vi "Setup UI.vi"(8 "error in (no error)":errorcluster, 10 "Set UI to input? (F)":bool, 11 "Wavelength iHR320 in":refnum<class "Wavelength ActiveX.lvclass">) -> (0 "error out":errorcluster, 3 "Wavelength iHR320 out":refnum<class "Wavelength ActiveX.lvclass">)   [LabVIEW 2023, in "Wavelength ActiveX.lvclass"]
doc: "Scanner::Setup is a constructor that has no parameters and faces the user. The Factory calls this VI to let the user configure this Scanner. It is dynamically dispatched in order to let the user choose the type as well as the options of the scanner."
uses:
  Wavelength ActiveX.lvclass
  Wavelength ActiveX.lvclass/Wavelength ActiveX.ctl
panel:
  in  "Select Filter":i32(ring)=1 items=["Filter 1"=1, "Empty"=2, "Empty"=3, "Empty"=4, "Filter 2"=5, "Filter 3"=6]
  out "Current Filter":i32(ring)=1 items=["Filter 1"=1, "Empty"=2, "Empty"=3, "Empty"=4, "Filter 2"=5, "Filter 3"=6]
  out "Current Position":dbl[unit]
  in  "GoTo First Step":bool
  out "Current Grating":dbl
  out "Step Size":dbl[unit]
  in  "Exit Slit":dbl[unit]=0.001
  in  "Entrance Slit":dbl[unit]=0.001
  in  "Override":bool
  in  "Select Grating":u16(ring)=2 items=["1200"=1, "600"=2]
  in  "Front Exit":dbl[unit]
  in  "Front Entrance":dbl[unit]
  # "iHR 320 Wavelength"
  # "lines/mm"
  # "lines/mm"
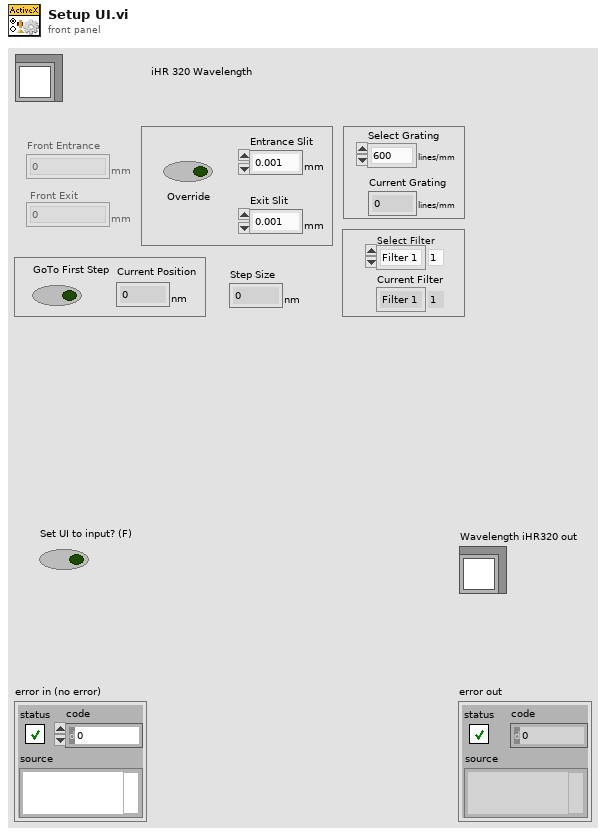
[diagram p1: front panel]
types:
  T1 = typedef "Scanner.lvclass/Range.ctl" = cluster{"xi":dbl, "xf":dbl, "dx":dbl, "Return to...?":bool, "Return to":dbl}
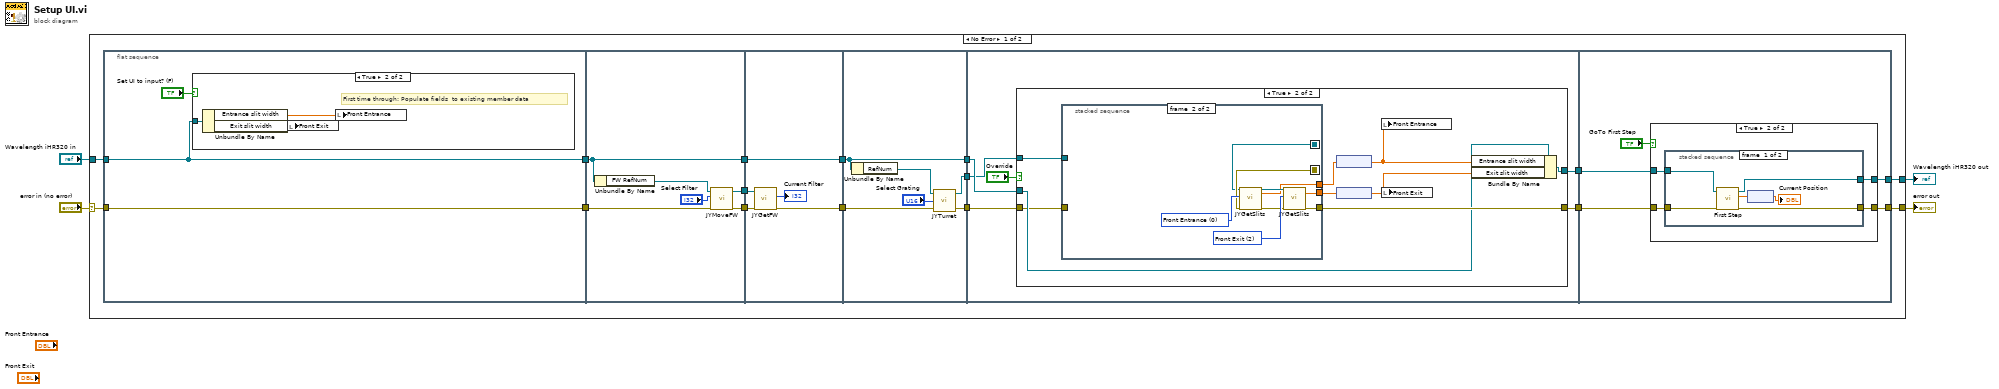
[diagram p0: block diagram]
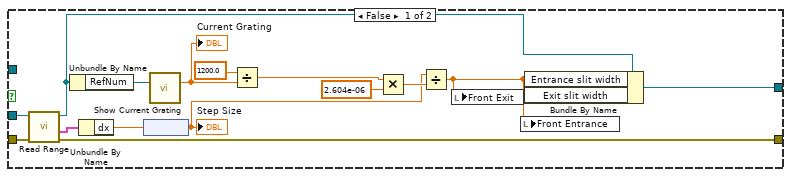
[diagram p3: hidden frame]
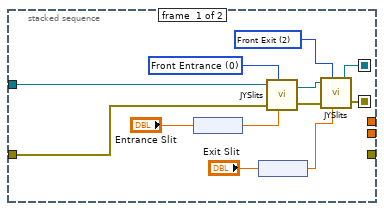
[diagram p4: hidden frame]
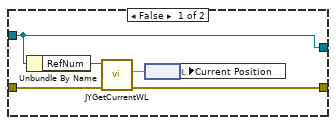
[diagram p5: hidden frame]
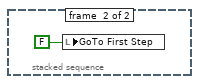
[diagram p6: hidden frame]
diagram:
  n1 = case shown="No Error" "error in (no error)" {
    selector: "error in (no error)" -> [w19 w118]
    tunnel: [w17 w118] -> w3
    tunnel: "Wavelength iHR320 in" -> [w20 w117]
    tunnel: [w18 w117] -> w1
    frame No Error {
      n2 = flat-sequence {
        tunnel: w20 -> [w21]
        tunnel: [w21] -> w12
        tunnel: [w22] -> w11
        tunnel: w19 -> [w22]
        tunnel: w12 -> [w29]
        tunnel: [w29] -> w10
        tunnel: w11 -> [w31]
        tunnel: [w30] -> w8
        tunnel: [w27] -> w6
        tunnel: w10 -> [w37]
        tunnel: [w37] -> w9
        tunnel: w8 -> [w35]
        tunnel: [w34] -> w7
        tunnel: w6 -> [w33]
        tunnel: w9 -> [w40]
        tunnel: w7 -> [w41]
        tunnel: [w40] -> w14
        tunnel: [w39] -> w13
        tunnel: [w38] -> w5
        tunnel: [w47] -> w16
        tunnel: [w48] -> w15
        tunnel: w14 -> [w46]
        tunnel: w13 -> [w45]
        tunnel: w5 -> [w44]
        tunnel: [w97] -> w17
        tunnel: [w96] -> w18
        tunnel: w16 -> [w99]
        tunnel: w15 -> [w98]
        frame #0 {
          n3 = case shown="True" "Set UI to input? (F)" {
            tunnel: w21 -> [_ w24]
            frame False {
              # "Subsequent times through: Populate member data  according to existing fields"
            }
            frame True {
              # "First time through: Populate fields  to existing member data"
              n4 = Unbundle By Name(w24) -> ("Entrance slit width"=w26:dbl[unit], "Exit slit width"=w25:dbl[unit])
              n5 = local write "Front Exit"(w25) -> ()
              n6 = local write "Front Entrance"(w26) -> ()
            }
          }
        }
        frame #1 {
          n7 = Unbundle By Name(w29) -> ("FW RefNum"=w28:refnum<k7>)
          n8 = call "JYMoveFW.vi"("error in (no error)"=w31, "Filter Index"="Select Filter", "FW RefNum In"=w28) -> ("error out"=w30:errorcluster, "FW RefNum Out"=w27:refnum<k7>)  [unwired: 7 in]
        }
        frame #2 {
          n9 = call "JYGetFW.vi"("error in (no error)"=w35, "FW RefNum In"=w33) -> ("error out"=w34:errorcluster, "Filter Index"=→"Current Filter":i32)  [unwired: 7 in, 1 out]
        }
        frame #3 {
          n10 = Unbundle By Name(w40) -> ("RefNum"=w42:refnum<k7>)
          n11 = call "JYTurret.vi"("error in (no error)"=w41, "Grating Index"="Select Grating", "JYMONOLib.IJYMonoReqd In"=w42) -> ("error out"=w39:errorcluster, "JYMONOLib.IJYMonoReqd Out"=w38:refnum<k7>)  [unwired: 1 out]
        }
        frame #4 {
          n12 = case shown="True" "Override" {
            tunnel: [w54 w73] -> w48
            tunnel: [w53 w72] -> w47
            tunnel: w46 -> [w51 w67]
            tunnel: w45 -> [w50 w66]
            tunnel: w44 -> [_ w65]
            frame False {
              n13 = call-dynamic "Read Range.vi"("error in (no error)"=w50, "Scanner.lvclass in"=w51) -> ("error out"=w54:errorcluster, "Range"=w52:T1, "Scanner.lvclass out"=w62:refnum<class "Wavelength ActiveX.lvclass">)  [unwired: 4 in, 3 out]
              n14 = Unbundle By Name(w62) -> ("RefNum"=w63:refnum<k7>)
              n15 = Unbundle By Name(w52) -> ("dx"=w64:dbl)
              n16 = node(w64) -> (w56:dbl[unit])
              "Step Size" <- w56
              n17 = call "Show Current Grating.vi"("JYMONOLib.IJYMonoReqd  in"=w63) -> ("Current Grating"=w60:dbl)  [unwired: 6 in, 8 out]
              "Current Grating" <- w60
              n18 = Divide(x=1200.0, y=w60) -> (x/y=w59:dbl)
              n19 = Multiply(x=w59, y=2.604e-06) -> (x*y=w57:dbl)
              n20 = Divide(x=w56, y=w57) -> (x/y=w55:dbl[unit])
              n21 = local write "Front Exit"(w55) -> ()
              n22 = local write "Front Entrance"(w55) -> ()
              n23 = Bundle By Name(cluster=w62, "Entrance slit width"=w55, "Exit slit width"=w55) -> (w53:refnum<class "Wavelength ActiveX.lvclass">)
            }
            frame True {
              n24 = stacked-sequence {
                seq-local: [w77 _] -> [_ w91]
                seq-local: [w74 _] -> [_ w86]
                tunnel: [_ w89] -> w73
                tunnel: [_ w88] -> w71
                tunnel: [_ w87] -> w70
                tunnel: w66 -> [w76 _]
                tunnel: w65 -> [w75 _]
                frame #0 {
                  w83 = u16 2 items=["Front Entrance", "Side Entrance", "Front Exit", "Side Exit", "First Intermediate", "Second Intermediate"] ("Slit")
                  w84 = u16 0 items=["Front Entrance", "Side Entrance", "Front Exit", "Side Exit", "First Intermediate", "Second Intermediate"] ("Slit")
                  n25 = node("Entrance Slit") -> (w85:dbl)
                  n26 = node("Exit Slit") -> (w82:dbl)
                  n27 = call "JYSlits.vi"("JYMONOLib.IJYMonoReqd In"=w75, "Slit"=w84, "error in (no error)"=w76, "Slit Width"=w85) -> ("JYMONOLib.IJYMonoReqd Out"=w81:refnum<k7>, "error out"=w80:errorcluster)  [unwired: 1 in]
                  n28 = call "JYSlits.vi"("JYMONOLib.IJYMonoReqd In"=w81, "Slit"=w83, "error in (no error)"=w80, "Slit Width"=w82) -> ("JYMONOLib.IJYMonoReqd Out"=w74:refnum<k7>, "error out"=w77:errorcluster)  [unwired: 1 in]
                }
                frame #1 {
                  w92 = u16 2 items=["Front Entrance", "Side Entrance", "Front Exit", "Side Exit", "First Intermediate", "Second Intermediate"] ("Slit")
                  w93 = u16 0 items=["Front Entrance", "Side Entrance", "Front Exit", "Side Exit", "First Intermediate", "Second Intermediate"] ("Slit")
                  n29 = call "JYGetSlits.vi"("MonoRefNum IN"=w86, "Slit"=w93, "error in (no error)"=w91) -> ("MonoRefNum Out"=w94:refnum<k7>, "Slit Width"=w88:dbl, "error out"=w90:errorcluster)  [unwired: 13 in, 1 out]
                  n30 = call "JYGetSlits.vi"("MonoRefNum IN"=w94, "Slit"=w92, "error in (no error)"=w90) -> ("Slit Width"=w87:dbl, "error out"=w89:errorcluster)  [unwired: 13 in, 2 out]
                }
              }
              n31 = node(w71) -> (w68:dbl[unit])
              n32 = node(w70) -> (w69:dbl[unit])
              n33 = local write "Front Entrance"(w68) -> ()
              n34 = local write "Front Exit"(w69) -> ()
              n35 = Bundle By Name(cluster=w67, "Entrance slit width"=w68, "Exit slit width"=w69) -> (w72:refnum<class "Wavelength ActiveX.lvclass">)
            }
          }
        }
        frame #5 {
          n36 = case shown="True" "GoTo First Step" {
            tunnel: w99 -> [w105 w109]
            tunnel: w98 -> [w103 w108]
            tunnel: [w102 w107] -> w97
            tunnel: [w105 w106] -> w96
            frame False {
              n37 = Unbundle By Name(w105) -> ("RefNum"=w104:refnum<k7>)
              n38 = call "JYGetCurrentWL.vi"("error in (no error)"=w103, "JYMONOLib.IJYMonoReqd In"=w104) -> ("error out"=w102:errorcluster, "Current WL"=w101:dbl)  [unwired: 6 in, 2 out]
              n39 = node(w101) -> (w100:dbl[unit])
              n40 = local write "Current Position"(w100) -> ()
            }
            frame True {
              n41 = stacked-sequence {
                tunnel: w109 -> [w115 _]
                tunnel: w108 -> [w114 _]
                tunnel: [w113 _] -> w107
                tunnel: [w112 _] -> w106
                frame #0 {
                  n42 = call-dynamic "First Step.vi"("error in (no error)"=w114, "Wavelength iHR320.lvclass in"=w115) -> ("error out"=w113:errorcluster, "Current Position"=w111:dbl, "Wavelength iHR320.lvclass out"=w112:refnum<class "Wavelength ActiveX.lvclass">)  [unwired: 7 in]
                  n43 = node(w111) -> (→"Current Position":dbl[unit])
                }
                frame #1 {
                  n44 = local write "GoTo First Step"(FALSE ("GoTo First Step")) -> ()
                }
              }
            }
          }
        }
      }
    }
    frame Error {
    }
  }
  "error out" <- w3
  "Wavelength iHR320 out" <- w1
